vi "ELVIS III v1.0 Unreserve DO Block.vi"(7 "Allow multiple opens?":bool, 8 "error in (no error)":errorcluster, 10 "DO (N Samples) Channel List":T2, 11 "Generic FPGA Reference":T1) -> (0 "error out":errorcluster)   [LabVIEW 2021]
uses:
  <vilib>/myRIO/Common/Instrument Driver Framework/myRIO v1.0/DO Block/typedefs/DO Block Channels List.ctl
  <vilib>/myRIO/Common/Instrument Driver Framework/myRIO v1.0/DO Block/typedefs/DO Block Channels Enum.ctl
  <vilib>/myRIO/Common/Instrument Driver Framework/Utilities/typedefs/Generic FPGA Reference.ctl
  <vilib>/myRIO/Common/Instrument Driver Framework/ELVIS III v1.0/Resource Manager/vis/ELVIS III v1.0 Create Configuration List.vi
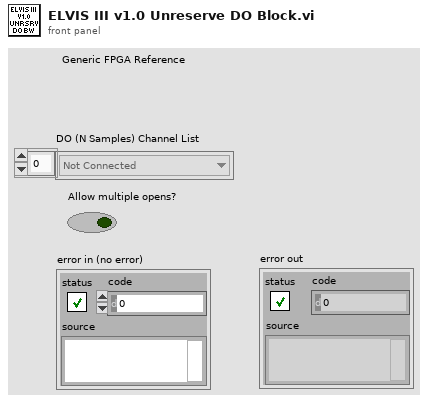
[diagram p1: front panel]
types:
  T1 = typedef "Generic FPGA Reference.ctl" = refnum<k20>
  T2 = typedef "DO Block Channels List.ctl" = T3[]
  T3 = typedef "DO Block Channels Enum.ctl" = enum16{"Not Connected", "A/DO0 (N Samples)", "A/DO1 (N Samples)", "A/DO2 (N Samples)", "A/DO3 (N Samples)", "A/DO4 (N Samples)", "A/DO5 (N Samples)", "A/DO6 (N Samples)", "A/DO7 (N Samples)", "A/DO8 (N Samples)", "A/DO9 (N Samples)", "A/DO10 (N Samples)", "A/DO11 (N Samples)", "A/DO12 (N Samples)", "A/DO13 (N Samples)", "A/DO14 (N Samples)", "A/DO15 (N Samples)", "A/DO16 (N Samples)", "A/DO17 (N Samples)", "A/DO18 (N Samples)", "A/DO19 (N Samples)", "B/DO0 (N Samples)", "B/DO1 (N Samples)", "B/DO2 (N Samples)", "B/DO3 (N Samples)", "B/DO4 (N Samples)", "B/DO5 (N Samples)", "B/DO6 (N Samples)", "B/DO7 (N Samples)", "B/DO8 (N Samples)", "B/DO9 (N Samples)", "B/DO10 (N Samples)", "B/DO11 (N Samples)", "B/DO12 (N Samples)", "B/DO13 (N Samples)", "B/DO14 (N Samples)", "B/DO15 (N Samples)", "B/DO16 (N Samples)", "B/DO17 (N Samples)", "B/DO18 (N Samples)", "B/DO19 (N Samples)"}
  T4 = typedef "ELVIS III v1.0 Channel Reservation List.ctl" = T5[]
  T5 = typedef "ELVIS III v1.0 Channel Reservation Info.ctl" = cluster{"Channel Name":string, "Connector":T6, "MutexIDs":u32[]}
  T6 = typedef "ELVIS III v1.0 Connector List.ctl" = enum32{"None", "ConnectorA", "ConnectorB"}
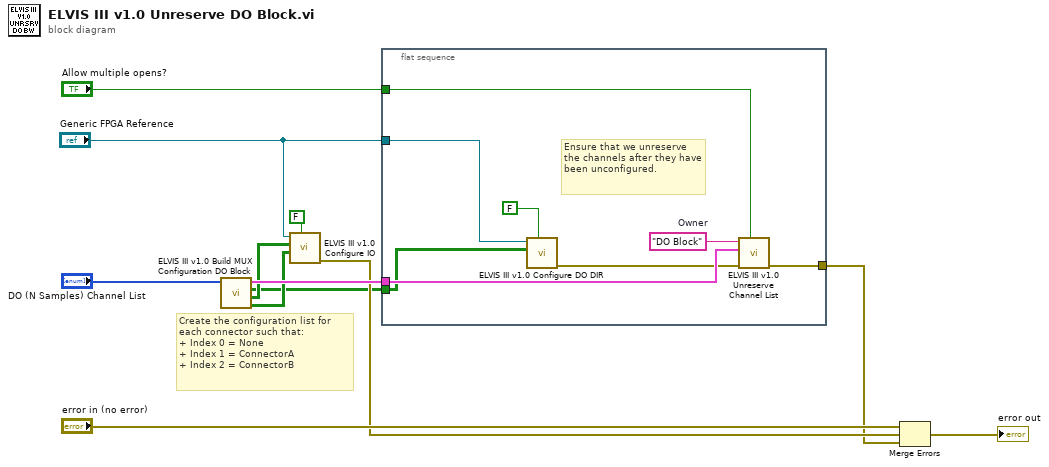
[diagram p0: block diagram]
diagram:
  # "Create the configuration list for each connector such that:\n+ Index 0 = None\n+ Index 1 = ConnectorA\n+ Index 2 = ConnectorB"
  n1 = call <vilib>:"ELVIS III v1.0 Build MUX Configuration DO Block.vi"("DO (N Samples) Channel List"="DO (N Samples) Channel List") -> ("Configuration Bitmask Array"=w5:bool[][], "Configration Bitcode Array"=w6:bool[][], "DIO Mode Bitmask"=w2:bool[][], "Channel Reservation List"=w9:T4)  [unwired: 7 in]
  n2 = call <vilib>:"ELVIS III v1.0 Configure IO.vi"("Value"=FALSE, "Bitmask Array"=w5, "Bitcode Array"=w6, "myRIO FPGA Ref In"="Generic FPGA Reference") -> ("error out"=w4:errorcluster)  [unwired: 7 in]
  n3 = flat-sequence {
    tunnel: "Allow multiple opens?" -> [w20]
    tunnel: w9 -> [w18]
    tunnel: [w17] -> w3
    tunnel: w2 -> [w16]
    tunnel: "Generic FPGA Reference" -> [w14]
    frame #0 {
      w19 = "DO Block"  # Owner
      # "Ensure that we unreserve the channels after they have been unconfigured."
      n4 = call <vilib>:"ELVIS III v1.0 Configure DO DIR.vi"("Apply Bitmask?"=FALSE, "Bitmask Array"=w16, "myRIO FPGA Ref In"=w14) -> ("error out"=w13:errorcluster)  [unwired: 8 in]
      n5 = call <vilib>:"ELVIS III v1.0 Unreserve Channel List.vi"("Allow multiple opens?"=w20, "error in (no error)"=w13, "Channel Reservation List"=w18, "Owner"=w19) -> ("error out"=w17:errorcluster)  [unwired: 7 in]
    }
  }
  n6 = Merge Errors("error in (no error)", w4, w3) -> (→"error out":errorcluster)
